vi "2D Matrix (Zeros).vi"(9 "element (0)":dbl format="%#_13g", 10 "nCols (1)":i32, 11 "nRows":i32) -> (3 "Real Matrix":T1)   [LabVIEW 2014]
uses:
  <vilib>/Analysis/Matrix/Datatypes/RealMatrix.ctl
  <vilib>/Analysis/Matrix/Numeric/Conversions/Array To Matrix - RA2.vi
  <vilib>/Analysis/Matrix/NI_Matrix.lvlib
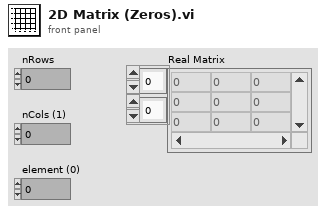
[diagram p1: front panel]
types:
  T1 = typedef "NI_Matrix.lvlib/RealMatrix.ctl" = dbl[][]
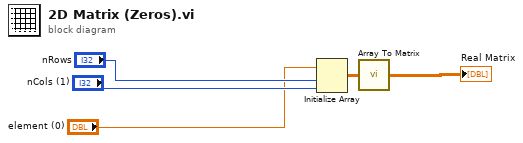
[diagram p0: block diagram]
diagram:
  n1 = Initialize Array("element (0)", "nRows", "nCols (1)") -> (w2:dbl[][])
  n2 = call-poly <vilib>:"Array To Matrix.vi"("Real 2D Array"=w2) -> ("Real Matrix"=→"Real Matrix":T1)
